vi "AlliGator Dispose Dataset Images.vi"(8 "Error In":errorcluster, 11 "Current Dataset Images 1":T1) -> (0 "Error Out":errorcluster, 3 "Gate Image Set":T1)   [LabVIEW 2021, in "AlliGator Files.lvlib"]
doc: "Disposes images corresponding to the loaded dataset."
uses:
  AlliGator Files.lvlib
  AlliGator Gate Image Set.ctl
  <vilib>/vision/Image Controls.llb/IMAQ Image.ctl
  Image/Image.lvlib
  AlliGator Internal Variables.lvlib
panel:
  # "see the AlliGator License on the block diagram (Ctrl+E or Window:Show Block Diagram)"
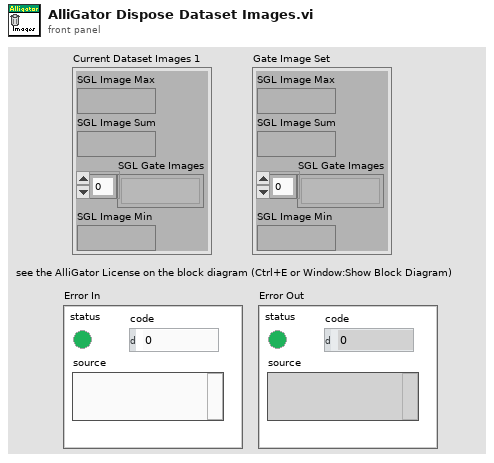
[diagram p1: front panel]
types:
  T1 = typedef "AlliGator Internal Variables.lvlib/AlliGator Gate Image Set.ctl" = cluster{"SGL Image Max":T2, "SGL Image Sum":T2, "SGL Gate Images":T2[], "SGL Image Min":T2}
  T2 = typedef "IMAQ Image.ctl" = refnum<image>
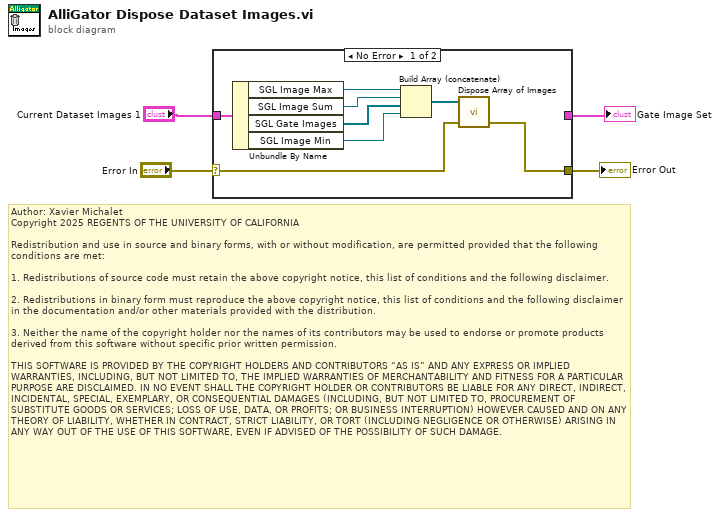
[diagram p0: block diagram]
diagram:
  # "Author: Xavier Michalet\nCopyright 2025 REGENTS OF THE UNIVERSITY OF CALIFORNIA\n\nRedistribution and use in source and binary forms, with or without modification, are permitted provided that the following conditions are met:\n\n1. Redistributions of source code must retain the above copyright notice, this list of conditions and the following disclaimer.\n\n2. Redistributions in binary form must reproduce the above copyright notice, this list of conditions and the following disclaimer in the documentation and/or other materials provided with the distribution.\n\n3. Neither the name of the copyright holder nor the names of its contributors may be used to endorse or promote products derived from this software without specific prior written permission.\n\nTHIS SOFTWARE IS PROVIDED BY THE COPYRIGHT HOLDERS AND CONTRIBUTORS “AS IS” AND ANY EXPRESS OR IMPLIED WARRANTIES, INCLUDING, BUT NOT LIMITED TO, THE IMPLIED WARRANTIES OF MERCHANTABILITY AND FITNESS FOR A PARTICULAR PURPOSE ARE DISCLAIMED. IN NO EVENT SHALL THE COPYRIGHT HOLDER OR CONTRIBUTORS BE LIABLE FOR ANY DIRECT, INDIRECT, INCIDENTAL, SPECIAL, EXEMPLARY, OR CONSEQUENTIAL DAMAGES (INCLUDING, BUT NOT LIMITED TO, PROCUREMENT OF SUBSTITUTE GOODS OR SERVICES; LOSS OF USE, DATA, OR PROFITS; OR BUSINESS INTERRUPTION) HOWEVER CAUSED AND ON ANY THEORY OF LIABILITY, WHETHER IN CONTRACT, STRICT LIABILITY, OR TORT (INCLUDING NEGLIGENCE OR OTHERWISE) ARISING IN ANY WAY OUT OF THE USE OF THIS SOFTWARE, EVEN IF ADVISED OF THE POSSIBILITY OF SUCH DAMAGE."
  n1 = case shown="No Error" "Error In" {
    selector: "Error In" -> [w6 w13]
    tunnel: "Current Dataset Images 1" -> [w12 w14]
    tunnel: [w5 w13] -> w2
    tunnel: [_ w14] -> w1
    frame No Error {
      n2 = Unbundle By Name(w12) -> ("SGL Image Max"=w11:T2, "SGL Image Sum"=w10:T2, "SGL Gate Images"=w9:T2[], "SGL Image Min"=w8:T2)
      n3 = Build Array (concatenate)(w11, w10, w9, w8) -> (w7:T2[])
      n4 = call "Dispose Array of Images.vi"("Array of Images"=w7, "error in (no error)"=w6) -> ("error out"=w5:errorcluster)  [unwired: 7 in]
    }
    frame Error {
    }
  }
  "Gate Image Set" <- w1
  "Error Out" <- w2
